vi "LineGetPoints (subVi).vi"(9 "Num Point":i32, 10 "End Point Coordinates":cluster{"X (m)":sgl, "Y (m)":sgl}={"X (m)"=-1.817262e-07, "Y (m)"=-2.0885543e-07}, 11 "Start Point Coordinates":cluster{"X (m)":sgl, "Y (m)":sgl}={"X (m)"=-1.817262e-07, "Y (m)"=-2.0885543e-07}) -> (3 "Array":cluster{"X (m)":sgl, "Y (m)":sgl}[](array[cluster]))   [LabVIEW 2014]
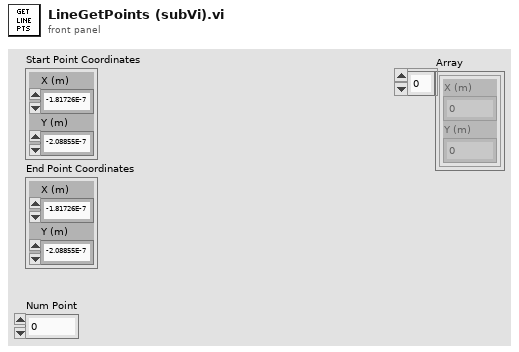
[diagram p1: front panel]
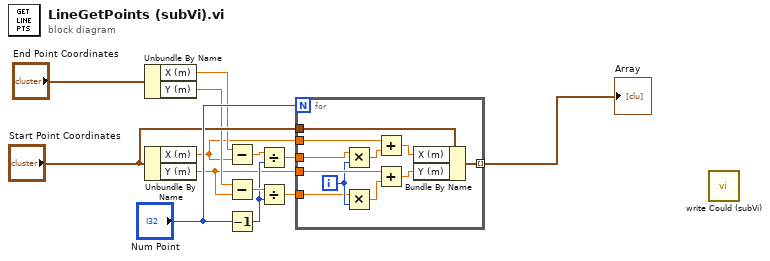
[diagram p0: block diagram]
diagram:
  n1 = Unbundle By Name("End Point Coordinates") -> ("X (m)"=w5:sgl, "Y (m)"=w4:sgl)
  n2 = Unbundle By Name("Start Point Coordinates") -> ("X (m)"=w2:sgl, "Y (m)"=w3:sgl)
  n3 = Subtract(x=w5, y=w2) -> (x-y=w12:sgl)
  n4 = Subtract(x=w4, y=w3) -> (x-y=w11:sgl)
  n5 = Decrement(x="Num Point") -> (x-1=w10:i32)
  n6 = Divide(x=w12, y=w10) -> (x/y=w8:sgl)
  n7 = Divide(x=w11, y=w10) -> (x/y=w7:sgl)
  n8 = for {
    N: "Num Point" -> [_]
    tunnel: w2 -> [w24]
    tunnel: w3 -> [w23]
    tunnel: w8 -> [w19]
    tunnel: w7 -> [w18]
    tunnel: "Start Point Coordinates" -> [w17]
    tunnel: [w14] -> w1 mode=indexing
    i -> [w20]
    n9 = Multiply(x=w19, y=w20) -> (x*y=w21:sgl)
    n10 = Multiply(x=w18, y=w20) -> (x*y=w22:sgl)
    n11 = Add(x=w24, y=w21) -> (x+y=w16:sgl)
    n12 = Add(x=w23, y=w22) -> (x+y=w15:sgl)
    n13 = Bundle By Name(cluster=w17, "X (m)"=w16, "Y (m)"=w15) -> (w14:cluster{"X (m)":sgl, "Y (m)":sgl})
  }
  "Array" <- w1
  n14 = call "write Could (subVi).vi"() -> ()  [unwired: 12 in]
